vi "db_transactions_delete.vi"(0 "UDL PATH IN":path, 1 "TABLE NAME":string, 2 "CONDITIONS":cluster{"FIELD":string, "VALUE":string}, 4 "MODE":bool, 5 "ERROR IN":errorcluster) -> (14 "UDL PATH OUT":path, 19 "ERROR OUT":errorcluster)   [LabVIEW 2018, in "db_lib R3.lvlib"]
uses:
  db_lib R3.lvlib
  <vilib>/addons/database/Connection.llb/DB Tools Open Connec (Path).vi
  <vilib>/addons/database/Connection.llb/Conn Execute.vi
  <vilib>/addons/database/Recordset.llb/Rec Destroy - Connection.vi
  <vilib>/addons/database/NI_Database_API.lvlib
panel:
  # "DELETE FROM [table_name] WHERE [condition]"
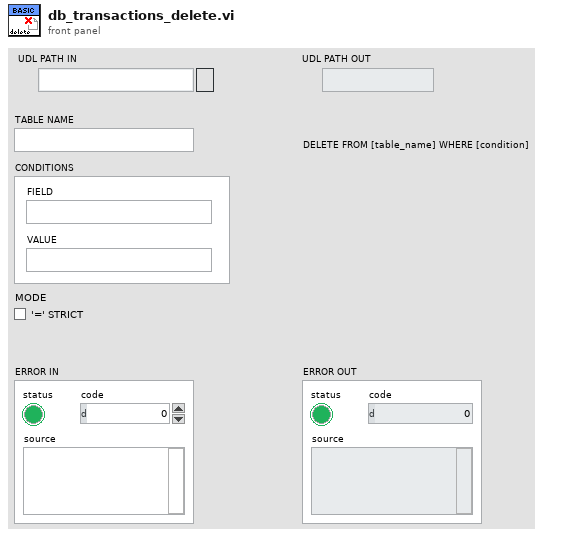
[diagram p1: front panel]
types:
  T1 = typedef "NI_Database_API.lvlib/Conn ObjectReference.ctl" = refnum<k1>
  T2 = typedef "NI_Database_API.lvlib/Rec ObjectReference.ctl" = refnum<k1>
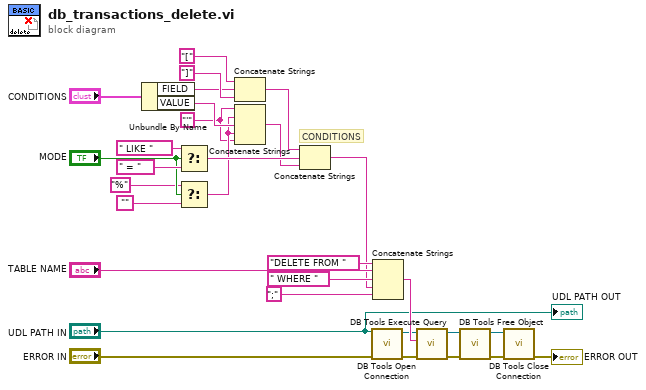
[diagram p0: block diagram]
diagram:
  w1 = "'" ("string")
  # "CONDITIONS"
  n1 = Unbundle By Name("CONDITIONS") -> ("FIELD"=w8:string, "VALUE"=w3:string)
  n2 = Select(t=" LIKE ", s="MODE", f=" = ") -> (s? t:f=w24:string)
  n3 = Select(t="%", s="MODE", f="") -> (s? t:f=w2:string)
  n4 = Concatenate Strings("[" ("string"), w8, "]" ("string")) -> (w11:string)
  n5 = Concatenate Strings(w1, w2, w3, w2, w1) -> (w10:string)
  n6 = Concatenate Strings(w11, w24, w10) -> (w7:string)
  n7 = call-poly <vilib>:"DB Tools Open Connection.vi"("error in (no error)"="ERROR IN", "connection information"="UDL PATH IN") -> ("error out"=w22:errorcluster, "connection reference"=w21:T1)  [unwired: 6 in]
  n8 = Concatenate Strings("DELETE FROM ", "TABLE NAME", " WHERE ", w7, ";" ("string")) -> (w28:string)
  n9 = call-poly <vilib>:"DB Tools Execute Query.vi"("error in (no error)"=w22, "SQL query"=w28, "connection reference"=w21) -> ("error out"=w27:errorcluster, "recordset reference"=w26:T2)  [unwired: 5 in]
  n10 = call-poly <vilib>:"DB Tools Free Object.vi"("error in (no error)"=w27, "recordset reference"=w26) -> ("error out"=w19:errorcluster, "connection reference"=w18:T1)  [unwired: 8 in]
  n11 = call <vilib>:"DB Tools Close Connection.vi"("error in (no error)"=w19, "connection reference"=w18) -> ("error out"=→"ERROR OUT":errorcluster)  [unwired: 5 in]
  "UDL PATH OUT" <- "UDL PATH IN"
